vi "Test_oven_ps.vi"() -> ()   [LabVIEW 2016]
panel:
  in  "Oven PS VISA resource":refnum<visa-resource-name>="TCPIP0::192.168.1.160::966::SOCKET"
  out "Oven PS read buffer":string
  in  "Loop multiple (ms) 2":u32=500
  out "Oven PS Iteration":i32
  in  "byte count 3":u32=15
  out "Oven PS Current Actual 2":dbl
  out "Oven PS Current Actual":i32(graph)
  out "Oven PS Voltage Actual 2":dbl
  out "Oven PS Voltage Actual":i32(graph)
  out "Oven PS Current Set":dbl
  out "Oven PS Voltage Set":dbl
  out "Oven PS Error":errorcluster
  in  "stop":bool
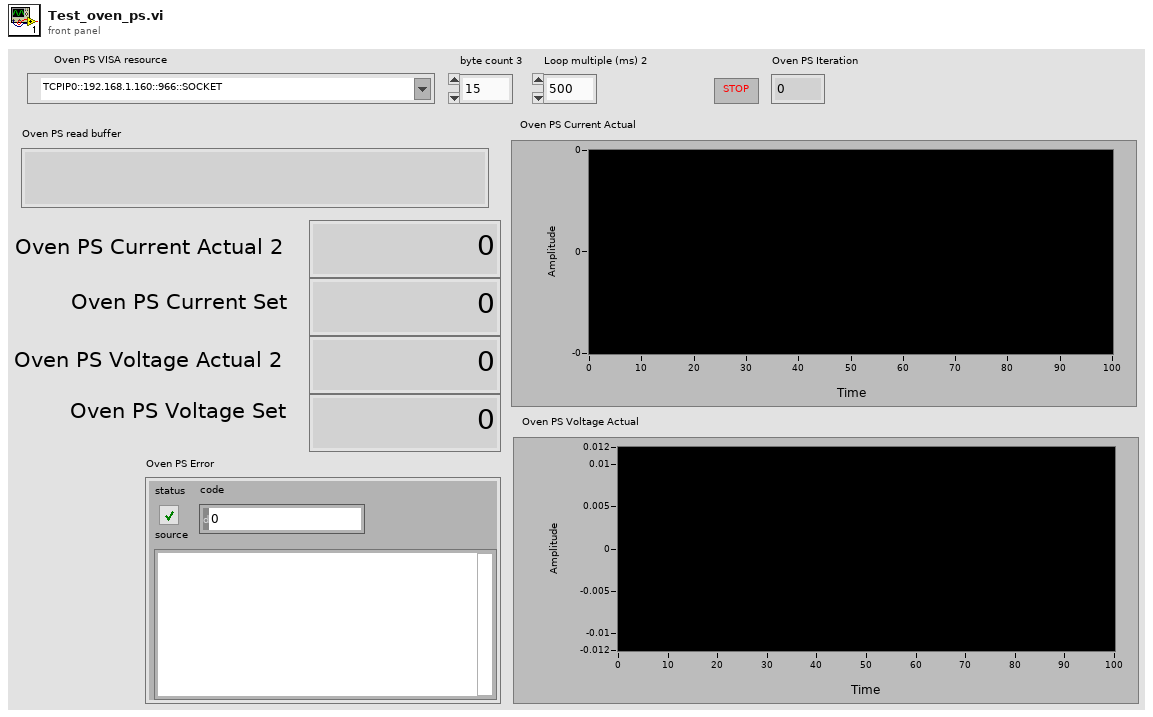
[diagram p1: front panel]
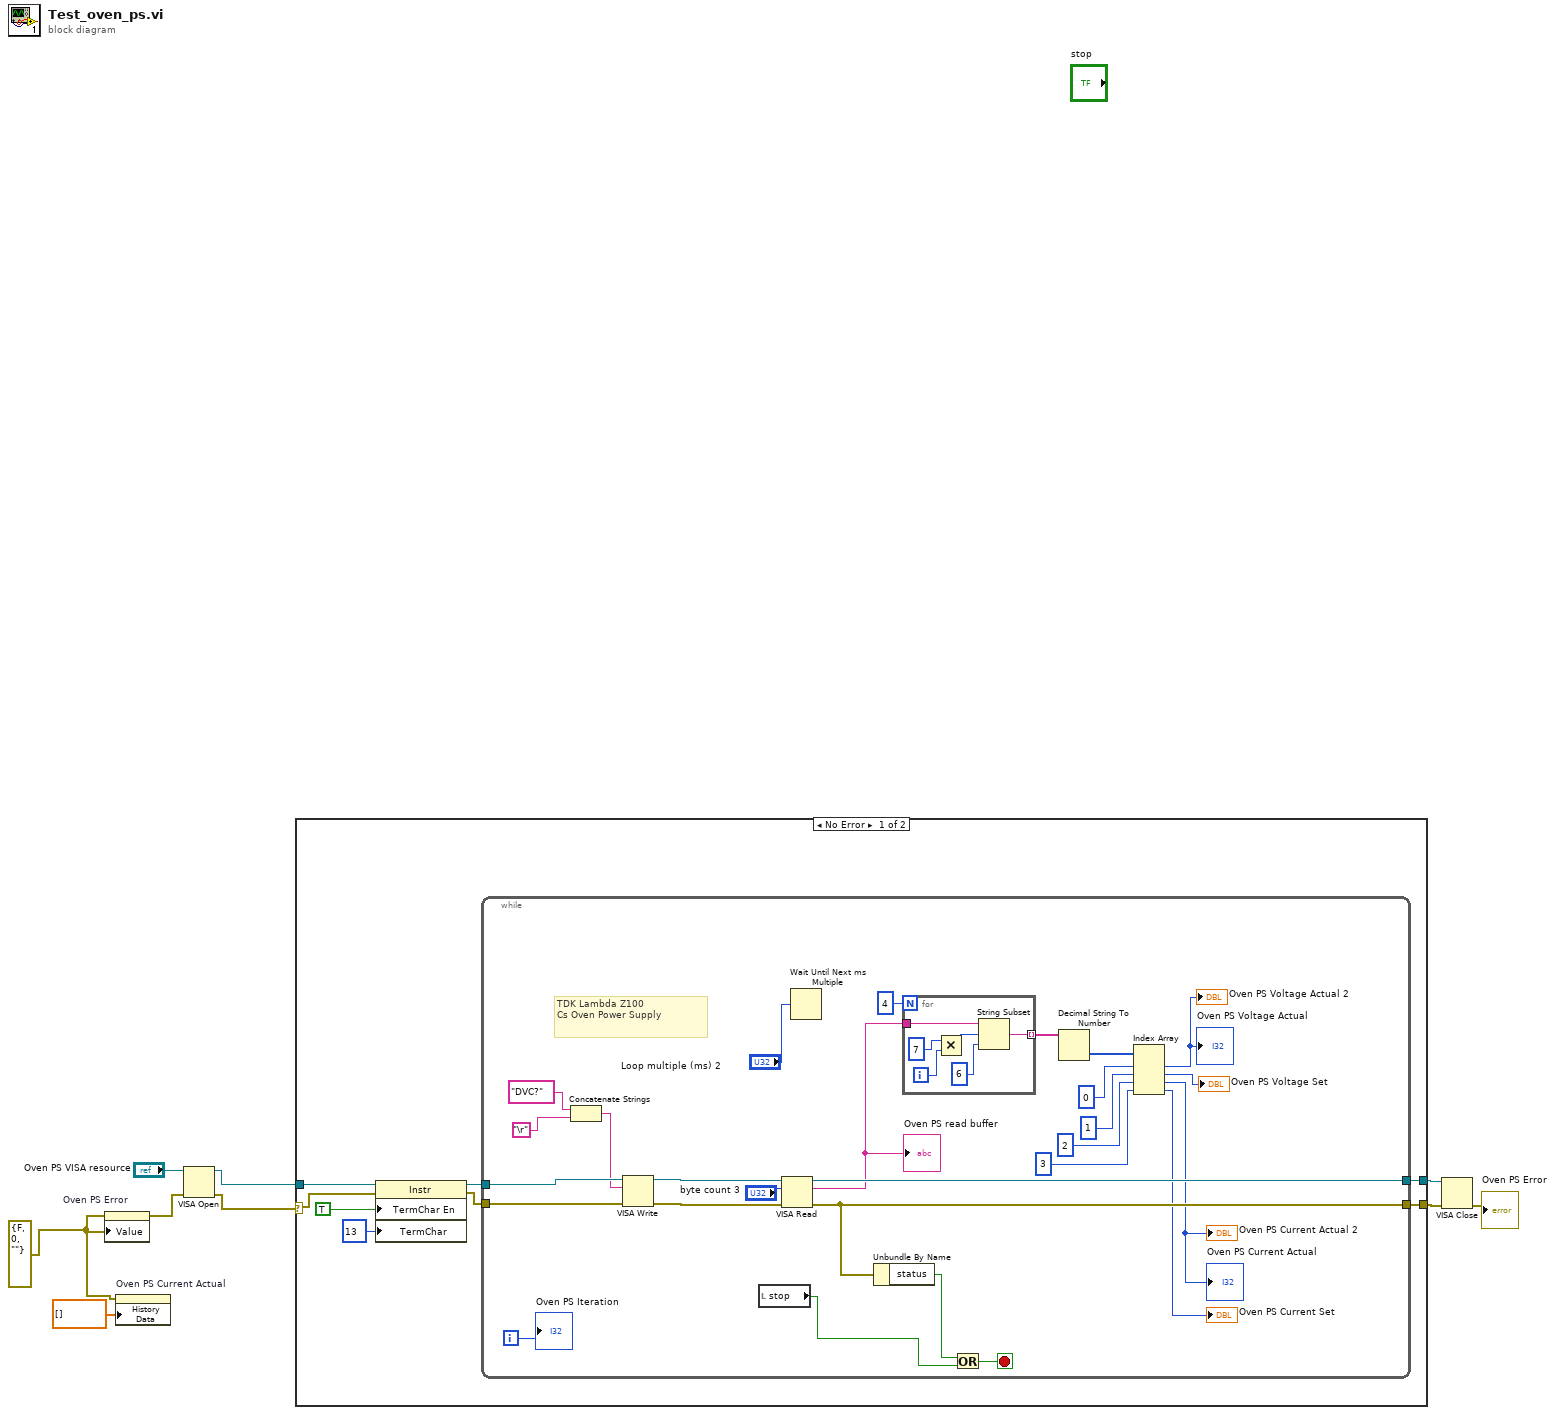
[diagram p0: block diagram]
diagram:
  w1 = errorcluster {"status"=FALSE, "code"=0, "source"=""} ("Oven PS Error")
  n1 = property on="Oven PS Error" class="Clust (strict)"(error in=w1, "Value"=w1) -> (error out=w5:errorcluster)  [unwired: 1 in, 1 out]
  n2 = property on="Oven PS Current Actual" class="WFChart (strict)"(error in=w1, "History Data"=dbl[] []) -> ()  [unwired: 1 in, 2 out]
  n3 = VISA Open(error in (no error)=w5, VISA resource name="Oven PS VISA resource") -> (VISA resource name=w9:refnum<visa-resource-name>, error out=w2:errorcluster)  [unwired: 3 in]
  n4 = case shown="No Error" w2 {
    selector: w2 -> [w10 w51]
    tunnel: w9 -> [w15 w52]
    tunnel: [w17 w52] -> w8
    tunnel: [w16 w51] -> w7
    frame No Error {
      n5 = property class="Instr"(reference=w15, error in=w10, "TermChar En"=TRUE ("Message Based Settings:Termination Character Enable"), "TermChar"=u8 13 ("Message Based Settings:Termination Character")) -> (reference out=w14:refnum<visa-resource-name>, error out=w13:errorcluster)
      n6 = while {
        tunnel: w14 -> [w35]
        tunnel: [w42] -> w17
        tunnel: w13 -> [w41]
        tunnel: [w39] -> w16
        i -> [w36]
        stop <- w37 stop-if-true
        # "TDK Lambda Z100\nCs Oven Power Supply"
        n7 = Concatenate Strings("DVC?" ("string"), "\r") -> (w31:string)
        n8 = VISA Write(VISA resource name=w35, write buffer=w31, error in (no error)=w41) -> (VISA resource name out=w43:refnum<visa-resource-name>, error out=w40:errorcluster)  [unwired: 1 out]
        n9 = local read "stop"() -> (w33:bool)
        n10 = VISA Read(VISA resource name=w43, byte count="byte count 3", error in (no error)=w40) -> (VISA resource name out=w42:refnum<visa-resource-name>, read buffer=w29:string, error out=w39:errorcluster)  [unwired: 1 out]
        "Oven PS read buffer" <- w29
        n11 = Wait Until Next ms Multiple(millisecond multiple="Loop multiple (ms) 2") -> ()  [unwired: 1 out]
        n12 = Unbundle By Name(w39) -> ("status"=w38:bool)
        n13 = for {
          N: 4 -> [_]
          tunnel: w29 -> [w50]
          tunnel: [w48] -> w19 mode=indexing
          i -> [w47]
          n14 = Multiply(x=7, y=w47) -> (x*y=w46:i32)
          n15 = String Subset(string=w50, offset (0)=w46, length (rest)=6 ("length (rest)")) -> (substring=w48:string)
        }
        n16 = Or(x=w38, y=w33) -> (x .or. y?=w37:bool)
        n17 = Decimal String To Number(string=w19) -> (number=w18:i32[])  [unwired: 2 in, 1 out]
        n18 = Index Array(array=w18, index #1=0 ("index"), index #2=1 ("index"), index #3=2 ("index"), index #4=3 ("index")) -> (element #1=→"Oven PS Voltage Actual 2" →"Oven PS Voltage Actual":i32, element #2=→"Oven PS Voltage Set":i32, element #3=→"Oven PS Current Actual 2" →"Oven PS Current Actual":i32, element #4=→"Oven PS Current Set":i32)
        "Oven PS Iteration" <- w36
      }
    }
    frame Error {
    }
  }
  n19 = VISA Close(VISA resource name=w8, error in (no error)=w7) -> (error out=→"Oven PS Error":errorcluster)
